vi "UpdateSoleNoid.vi"(8 "error in (no error)":errorcluster, 10 "Boolean":bool, 11 "ParameterConf in":refnum<class "ParameterConf.lvclass">) -> (0 "error out":errorcluster, 3 "ParameterConf out":refnum<class "ParameterConf.lvclass">)   [LabVIEW 2017, in "LibraryGcode.lvlib" / "ParameterConf.lvclass"]
uses:
  ParameterConf.lvclass
  ParameterConf.lvclass/ParameterConf.ctl
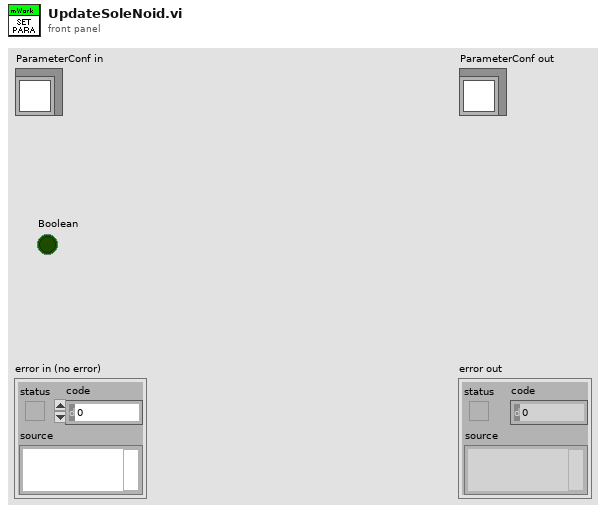
[diagram p1: front panel]
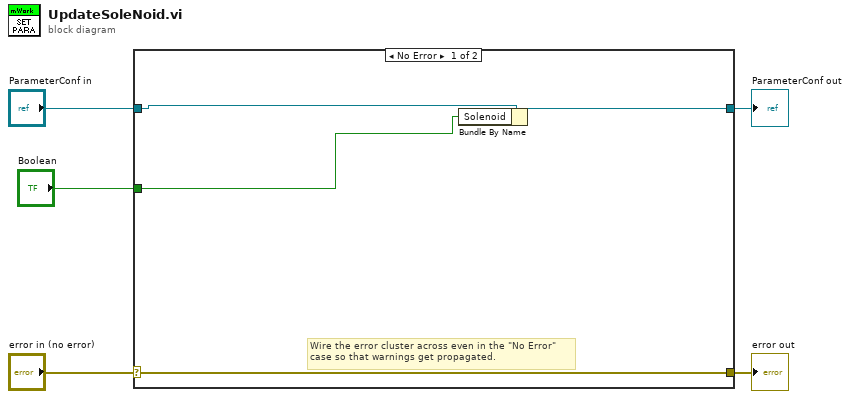
[diagram p0: block diagram]
diagram:
  n1 = case shown="No Error" "error in (no error)" {
    selector: "error in (no error)" -> [w9 w11]
    tunnel: [w9 w11] -> w4
    tunnel: [w7 w10] -> w2
    tunnel: "ParameterConf in" -> [w8 w10]
    tunnel: "Boolean" -> [w6 _]
    frame No Error {
      # "Wire the error cluster across even in the \"No Error\"\ncase so that warnings get propagated."
      n2 = Bundle By Name(cluster=w8, "Solenoid"=w6) -> (w7:refnum<class "ParameterConf.lvclass">)
    }
    frame Error {
    }
  }
  "error out" <- w4
  "ParameterConf out" <- w2
